vi "Begin.vi"(8 "error in (no error)":errorcluster, 11 "FileConfig in":refnum<class "FileConfig.lvclass">) -> (0 "error out":errorcluster, 3 "FileConfig out":refnum<class "FileConfig.lvclass">, 5 "File Found?":bool)   [LabVIEW 2019, in "Config.lvlib" / "FileConfig.lvclass"]
uses:
  FileConfig.lvclass
  FileConfig.lvclass/FileConfig.ctl
  Config.lvclass
  <vilib>/Utility/config.llb/NI_LVConfig.lvlib
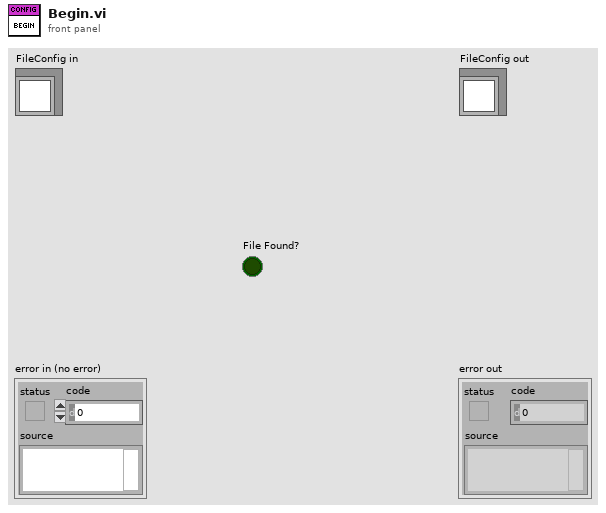
[diagram p1: front panel]
types:
  T1 = typedef "NI_LVConfig.lvlib/Config Data RefNum.ctl" = refnum<k1>
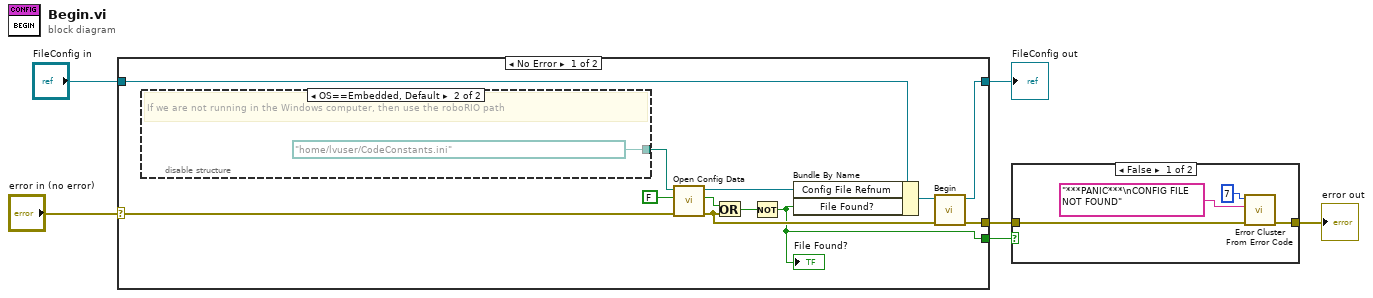
[diagram p0: block diagram]
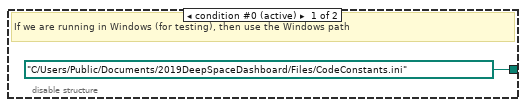
[diagram p3: hidden frame]
diagram:
  n1 = case shown="No Error" "error in (no error)" {
    selector: "error in (no error)" -> [w15 w22]
    tunnel: [w13 w22] -> w2
    tunnel: [w17 w21] -> w4
    tunnel: "FileConfig in" -> [w18 w21]
    tunnel: [w7 _] -> w3
    frame No Error {
      n2 = disable-structure shown="OS==Embedded, Default" {
        disable-tunnel: [path "C:/Users/Public/Documents/2019DeepSpaceDashboard/Files/CodeConstants.ini" ("configuration file path") path "/home/lvuser/CodeConstants.ini" ("configuration file path")] -> w8
        frame condition #0 (active) {
          # "If we are running in Windows (for testing), then use the Windows path"
        }
        frame condition #1 {
          # "If we are not running in the Windows computer, then use the roboRIO path"
        }
      }
      n3 = call <vilib>:"Open Config Data.vi"("error in (no error)"=w15, "create file if necessary (T)"=FALSE, "configuration file path"=w8) -> ("error out"=w10:errorcluster, "file created?"=w11:bool, "refnum"=w14:T1)  [unwired: 6 in]
      n4 = Or(x=w11, y=w10) -> (x .or. y?=w9:bool)
      n5 = Not(x=w9) -> (.not. x?=w7:bool)
      "File Found?" <- w7
      n6 = Bundle By Name(cluster=w18, "Config File Refnum"=w14, "File Found?"=w7) -> (w12:refnum<class "FileConfig.lvclass">)
      n7 = call-parent "Begin.vi"("error in (no error)"=w10, "Config in"=w12) -> ("error out"=w13:errorcluster, "Config out"=w17:refnum<class "FileConfig.lvclass">)  [unwired: 7 in, 1 out]
    }
    frame Error {
    }
  }
  "FileConfig out" <- w4
  n8 = case shown="False" w3 {
    tunnel: w2 -> [w24 w27]
    tunnel: [w23 w27] -> w1
    frame False {
      n9 = call <vilib>:"Error Cluster From Error Code.vi"("error in (no error)"=w24, "error message (\"\")"="***PANIC***\nCONFIG FILE NOT FOUND" ("error message (\"\")"), "error code (0)"=7) -> ("error out"=w23:errorcluster)  [unwired: 6 in]
    }
    frame True {
    }
  }
  "error out" <- w1
